vi "Log Message.vi"(2 "message":string, 3 "Type":enum16{"Error", "Warning", "Note"}(ring)) -> ()   [LabVIEW 2016]
doc: "Write a message to a log file along with the current date and time."
uses:
  <vilib>/Utility/config.llb/Read Key (Path).vi
  <vilib>/Utility/config.llb/NI_LVConfig.lvlib
panel:
  out "log path":path
  out "config path":path
  out "time string":string
  out "date string":string
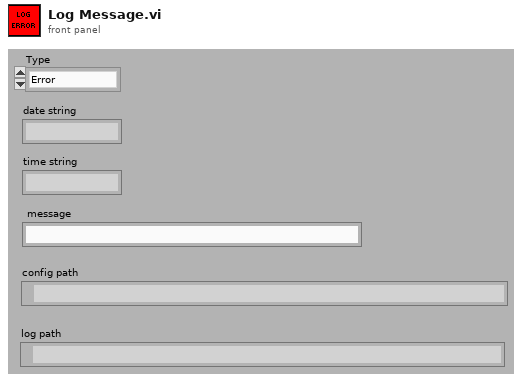
[diagram p1: front panel]
types:
  T1 = enum16{"open", "replace", "create", "open or create", "replace or create", "replace or create with confirmation"}
  T2 = typedef "NI_LVConfig.lvlib/Config Data RefNum.ctl" = refnum<k1>
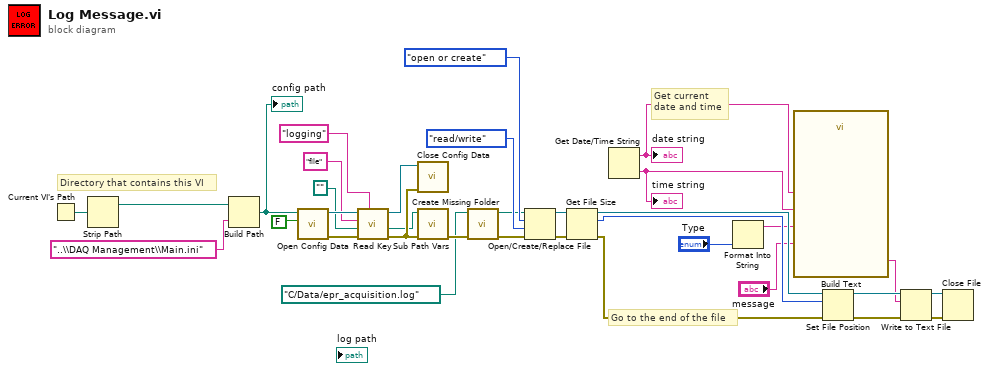
[diagram p0: block diagram]
diagram:
  # "Directory that contains this VI"
  # "Get current\ndate and time"
  # "Go to the end of the file"
  n1 = Current VI's Path() -> (path=w11:path)
  n2 = Strip Path(path=w11) -> (stripped path=w12:path)  [unwired: 1 out]
  n3 = Build Path(base path=w12, name or relative path="..\\DAQ Management\\Main.ini") -> (appended path=w15:path)
  "config path" <- w15
  n4 = call <vilib>:"Open Config Data.vi"("create file if necessary (T)"=FALSE, "configuration file path"=w15) -> ("error out"=w33:errorcluster, "refnum"=w32:T2)  [unwired: 7 in, 1 out]
  n5 = call-poly <vilib>:"Read Key.vi"("section"="logging", "error in (no error)"=w33, "default value"=path "", "key"="file", "refnum"=w32) -> ("error out"=w9:errorcluster, "value"=w8:path, "refnum out"=w29:T2)  [unwired: 3 in, 1 out]
  n6 = call <vilib>:"Close Config Data.vi"("error in (no error)"=w9, "refnum"=w29) -> ()  [unwired: 8 in, 2 out]
  n7 = call "Sub Path Vars.vi"("error in (no error)"=w9, "path"=w8) -> ("error out"=w7:errorcluster)  [unwired: 8 in, 1 out]
  n8 = call "Create Missing Folder.vi"("error in"=w7, "path"=path "C:/Data/epr_acquisition.log" ("abs path")) -> ("error out"=w6:errorcluster, "path dup"=w5:path)  [unwired: 7 in, 1 out]
  n9 = Open/Create/Replace File(file path (use dialog)=w5, error in=w6, operation (0:open)=T1."open or create", access (0:read/write)=enum16{"read/write", "read-only", "write-only"}."read/write") -> (refnum out=w28:refnum<file>, error out=w27:errorcluster)  [unwired: 2 in, 1 out]
  n10 = Get File Size(file=w28, error in=w27) -> (refnum out=w26:refnum<file>, size (in bytes)=w25:i64, 0:w24:errorcluster)
  n11 = Get Date/Time String() -> (date string=w18:string, time string=w19:string)  [unwired: 3 in]
  "date string" <- w18
  "time string" <- w19
  n12 = Format Into String("Type") -> (resulting string=w2:string)  [unwired: 3 in, 1 out]
  n13 = call "Build Text"("message"="message", "date"=w18, "time"=w19, "type"=w2) -> ("Result"=w17:string)  [unwired: 10 in, 1 out]
  n14 = Set File Position(offset (in bytes) (0)=w25, refnum=w26, error in=w24) -> (refnum out=w20:refnum<file>, error out=w23:errorcluster)  [unwired: 1 in]
  n15 = Write to Text File(file (use dialog)=w20, text=w17, error in=w23) -> (refnum out=w21:refnum<file>, error out=w22:errorcluster)  [unwired: 1 in, 1 out]
  n16 = Close File(refnum=w21, error in=w22) -> ()  [unwired: 2 out]
